vi "Tower light.vi"(10 "Enum":enum16{"Green", "Red", "Yellow", "OFF"}(ring)) -> ()   [LabVIEW 2020]
uses:
  Galobal variable_TI.vi
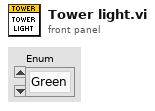
[diagram p1: front panel]
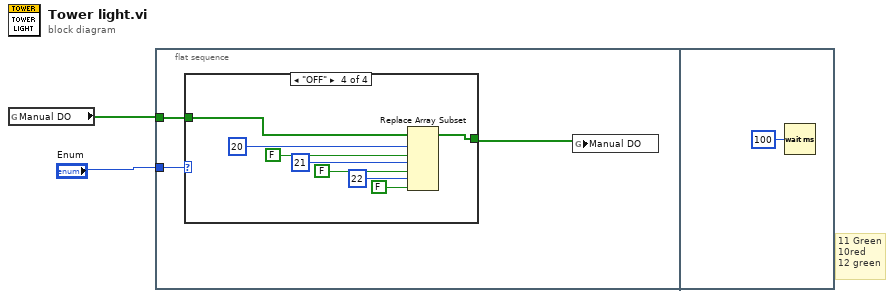
[diagram p0: block diagram]
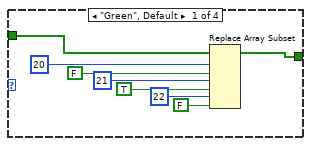
[diagram p2: hidden frame]
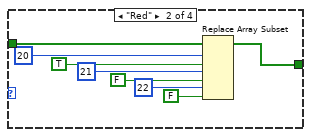
[diagram p3: hidden frame]
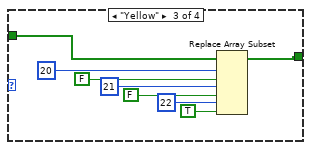
[diagram p4: hidden frame]
diagram:
  # "11 Green\n10red\n12 green"
  n1 = global read "Galobal variable_TI.vi" "Manual DO"() -> (w1:bool[])
  n2 = flat-sequence {
    tunnel: w1 -> [w5]
    tunnel: "Enum" -> [w4]
    frame #0 {
      n3 = case shown="\"OFF\"" w4 {
        tunnel: w5 -> [w7 w17 w23 w31]
        tunnel: [w6 w14 w22 w30] -> w3
        frame "Green", Default {
          n4 = Replace Array Subset(array=w7, new element #1=FALSE ("new element/subarray"), index #1=20 ("index"), new element #2=TRUE ("new element/subarray"), index #2=21 ("index"), new element #3=FALSE ("new element/subarray"), index #3=22 ("index")) -> (w6:bool[])
        }
        frame "Red" {
          n5 = Replace Array Subset(array=w17, new element #1=TRUE ("new element/subarray"), index #1=20 ("index"), new element #2=FALSE ("new element/subarray"), index #2=21 ("index"), new element #3=FALSE ("new element/subarray"), index #3=22 ("index")) -> (w14:bool[])
        }
        frame "Yellow" {
          n6 = Replace Array Subset(array=w23, new element #1=FALSE ("new element/subarray"), index #1=20 ("index"), new element #2=FALSE ("new element/subarray"), index #2=21 ("index"), new element #3=TRUE ("new element/subarray"), index #3=22 ("index")) -> (w22:bool[])
        }
        frame "OFF" {
          n7 = Replace Array Subset(array=w31, new element #1=FALSE ("new element/subarray"), index #1=20 ("index"), new element #2=FALSE ("new element/subarray"), index #2=21 ("index"), new element #3=FALSE ("new element/subarray"), index #3=22 ("index")) -> (w30:bool[])
        }
      }
      n8 = global write "Galobal variable_TI.vi" "Manual DO"(w3) -> ()
    }
    frame #1 {
      n9 = Wait (ms)(milliseconds to wait=u32 100) -> ()  [unwired: 1 out]
    }
  }
